vi "Draw.vi"(0 "reference in":refnum<class "Object.lvclass">, 1 "PictureIn":picture, 5 "error in (no error)":errorcluster) -> (14 "reference out":refnum<class "Object.lvclass">, 15 "PictureOut":picture, 19 "error out":errorcluster)   [LabVIEW 2019, in "Object.lvclass"]
doc: "Draws the Object/Creature"
uses:
  Object.lvclass
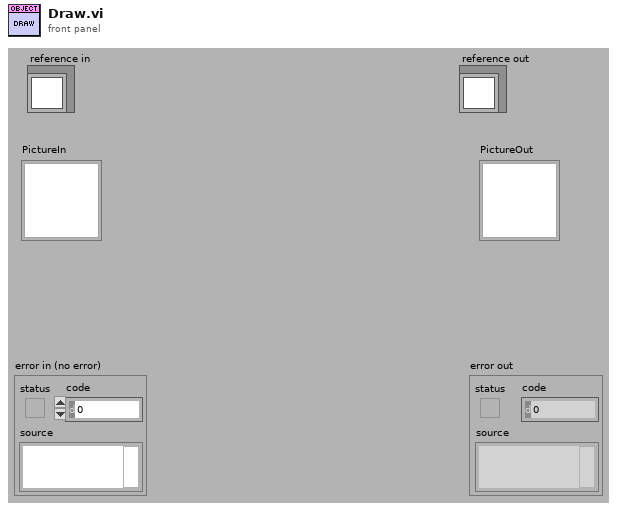
[diagram p1: front panel]
types:
  T1 = cluster{"left":i16, "top":i16, "right":i16, "bottom":i16}
  T2 = typedef "Object.lvclass/ObjectAttributes.ctl" = cluster{"X":i32, "y":i32, "Heading":enum16{"N", "E", "S", "W"}, "Map":refnum<class "Map.lvclass">, "MovementDelay":i32, "Color":u32}
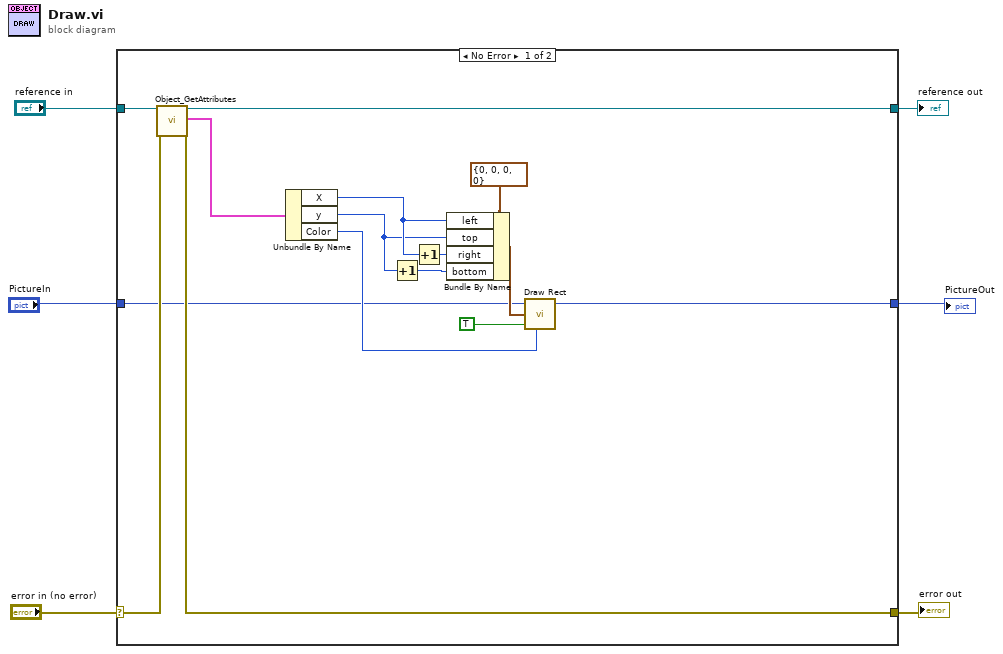
[diagram p0: block diagram]
diagram:
  n1 = case shown="No Error" "error in (no error)" {
    selector: "error in (no error)" -> [w21 w24]
    tunnel: [w20 w24] -> w5
    tunnel: [w18 w23] -> w3
    tunnel: "reference in" -> [w19 w23]
    tunnel: "PictureIn" -> [w8 w22]
    tunnel: [w7 w22] -> w1
    frame No Error {
      n2 = call "Object_GetAttributes.vi"("reference in"=w19, "error in (no error)"=w21) -> ("reference out"=w18:refnum<class "Object.lvclass">, "Attributes"=w9:T2, "error out"=w20:errorcluster)  [unwired: 15 out]
      n3 = Unbundle By Name(w9) -> ("X"=w15:i32, "y"=w14:i32, "Color"=w17:u32)
      n4 = Increment(x=w14) -> (x+1=w12:i32)
      n5 = Increment(x=w15) -> (x+1=w13:i32)
      n6 = Bundle By Name(cluster=T1 {"left"=0, "top"=0, "right"=0, "bottom"=0} ("rect"), "left"=w15, "top"=w14, "right"=w13, "bottom"=w12) -> (w11:T1)
      n7 = call <vilib>:"Draw Rect.vi"("picture"=w8, "rect"=w11, "fill?(F)"=TRUE, "color(black)"=w17) -> ("new picture"=w7:picture)  [unwired: 1 in, 4 out]
    }
    frame Error {
    }
  }
  "error out" <- w5
  "reference out" <- w3
  "PictureOut" <- w1
